vi "replaceUnsupportedChars.vi"(11 "stringIn":string) -> (2 "replaced?":bool, 3 "stringOut":string)   [LabVIEW 2023]
uses:
  <vilib>/Utility/error.llb/Trim Whitespace One-Sided.vi
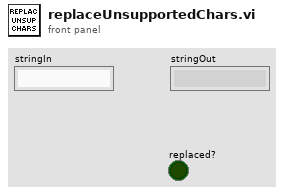
[diagram p1: front panel]
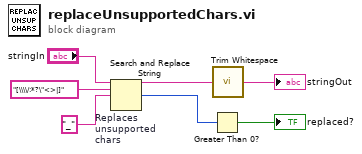
[diagram p0: block diagram]
diagram:
  n1 = Search and Replace String "Replaces\nunsupported\nchars"(input string="stringIn", search string="[\\\\/:*?\"<>|]", replace string="_" ("replace string (\"\")")) -> (result string=w7:string, number of replacements=w2:i32)  [unwired: 5 in, 2 out]
  n2 = Greater Than 0?(x=w2) -> (x > 0?=→"replaced?":bool)
  n3 = call <vilib>:"Trim Whitespace.vi"("string"=w7) -> ("trimmed string"=→"stringOut":string)  [unwired: 1 in]
